vi "Sub_Build_MQTT_String.vi"(8 "error in (no error)":errorcluster, 10 "String to be encoded":string="MQIsdp") -> (0 "error out":errorcluster, 2 "UTF8 Byte Array":u8[](array[numeric]) format="%x")   [LabVIEW 2012, in "MQTT_Functions.lvlib"]
uses:
  MQTT_Functions.lvlib
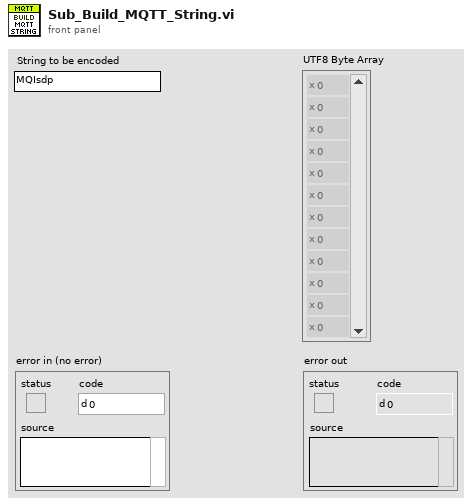
[diagram p1: front panel]
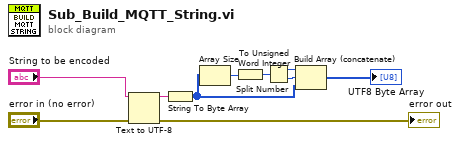
[diagram p0: block diagram]
diagram:
  n1 = Text to UTF-8(8:"error in (no error)", 11:"String to be encoded") -> (0:→"error out":errorcluster, 3:w8:string)
  n2 = String To Byte Array(string=w8) -> (unsigned byte array=w7:u8[])
  n3 = Array Size(array=w7) -> (size(s)=w6:i32)
  n4 = To Unsigned Word Integer(number=w6) -> (unsigned 16bit integer=w2:u16)
  n5 = Split Number(x=w2) -> (hi(x)=w4:u8, lo(x)=w5:u8)
  n6 = Build Array (concatenate)(w4, w5, w7) -> (→"UTF8 Byte Array":u8[])
